vi "Create log file.vi"(8 "error in (no error)":errorcluster) -> (0 "error out":errorcluster, 3 "log path":path)   [LabVIEW 2015]
uses:
  <vilib>/Utility/file.llb/Write Delimited Spreadsheet (string).vi
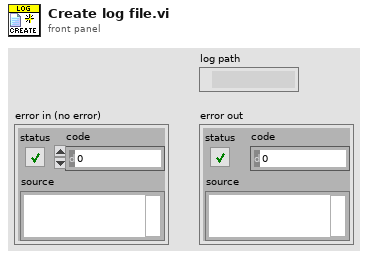
[diagram p1: front panel]
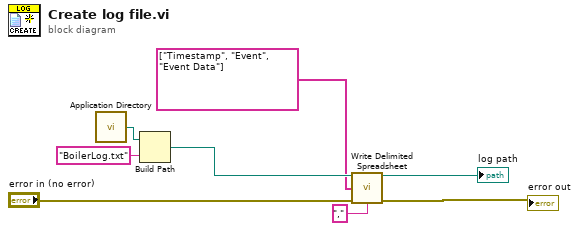
[diagram p0: block diagram]
diagram:
  n1 = call <vilib>:"Application Directory.vi"() -> ("Application Directory"=w7:path)
  n2 = Build Path(base path=w7, name or relative path="BoilerLog.txt") -> (appended path=w6:path)
  n3 = call-poly <vilib>:"Write Delimited Spreadsheet.vi"("file path (dialog if empty)"=w6, "1D data"=string[] ["Timestamp", "Event", "Event Data"], "error in (no error)"="error in (no error)", "delimiter (\\t)"="," ("delimiter (\\t)")) -> ("new file path (Not A Path if cancelled)"=→"log path":path, "error out"=→"error out":errorcluster)  [unwired: 10 in]
